vi "Count Pattern Frequencies.vi"(10 "Order":i32=1, 11 "File Data Array":T1[](array[typedef])) -> (3 "Pattern Frequencies":map{string[], i32}(c390))   [LabVIEW 2020]
uses:
  <vilib>/Utility/miscctls.llb/LVMapReplaceAction.ctl
  File Metadata.ctl
  Node.ctl
  Source to Sink Array.ctl
  File Data.ctl
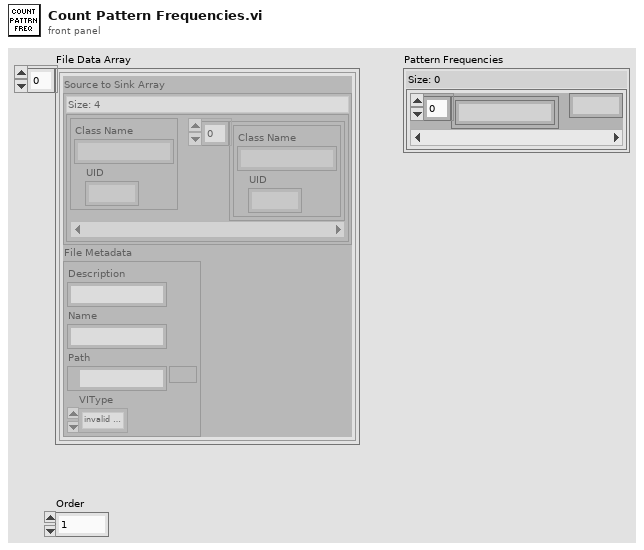
[diagram p1: front panel]
types:
  T1 = typedef "File Data.ctl" = cluster{"Source to Sink Array":T2, "File Metadata":T4}
  T2 = typedef "Source to Sink Array.ctl" = map{T3, T3[]}
  T3 = typedef "Node.ctl" = cluster{"Class Name":string, "UID":i32}
  T4 = typedef "File Metadata.ctl" = cluster{"Description":string, "Name":string, "Path":path, "VIType":enum32{"invalid VI type", "Standard VI", "Control VI", "Global VI", "Polymorphic VI", "Configuration VI", "SubSystem", "Facade VI", "Method VI", "Statechart Diagram VI"}}
  T5 = typedef "LVMapReplaceAction.ctl" = enum32{"Modify Entry only if found", "Add or Modify Entry", "Delete Entry"}
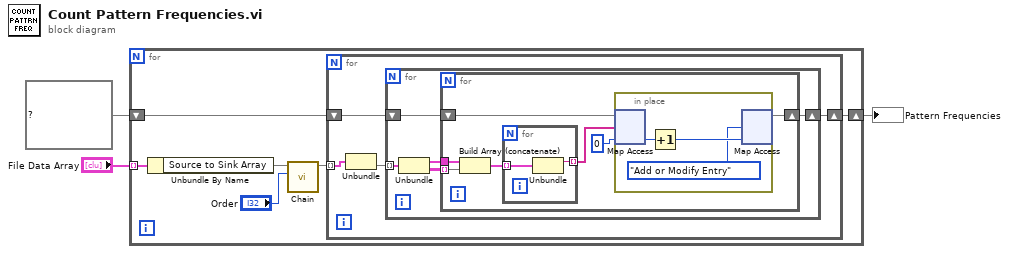
[diagram p0: block diagram]
diagram:
  n1 = for {
    shift-right: [w8] -> w3
    shift-left: map{string[], i32} {} ("Pattern Frequencies") -> [w9]
    tunnel: "File Data Array" -> [w5] mode=indexing
    n2 = Unbundle By Name(w5) -> ("Source to Sink Array"=w4:T2)
    n3 = call "Chain.vi"("Order"="Order", "Source to Sink Array"=w4) -> ("Node to Order-Length Paths"=w6:map{i32, map{T3, T3[][]}})  [unwired: 9 in]
    n4 = for {
      tunnel: w6 -> [w11] mode=indexing
      shift-right: [w12] -> w8
      shift-left: w9 -> [w13]
      n5 = Unbundle(w11) -> ("Source to Sink Array"=w10:map{T3, T3[][]})  [unwired: 1 out]
      n6 = for {
        tunnel: w10 -> [w18] mode=indexing
        shift-right: [w14] -> w12
        shift-left: w13 -> [w15]
        n7 = Unbundle(w18) -> ("Source"=w17:T3, "Sinks"=w16:T3[][])
        n8 = for {
          tunnel: w17 -> [w25]
          tunnel: w16 -> [w24] mode=indexing
          shift-right: [w19] -> w14
          shift-left: w15 -> [w20]
          n9 = Build Array (concatenate)(w25, w24) -> (w23:T3[])
          n10 = for {
            tunnel: w23 -> [w30] mode=indexing
            tunnel: [w29] -> w22 mode=indexing
            n11 = Unbundle(w30) -> ("Class Name"=w29:string)  [unwired: 1 out]
          }
          n12 = in-place {
            n13 = in-place-map #1(w20, w22, 0) -> (w28:i32)  [unwired: 1 out]
            n14 = Increment(x=w28) -> (x+1=w27:i32)
            n15 = in-place-map #1(w27, LVMapReplaceAction."Add or Modify Entry" ("action")) -> (w19:map{string[], i32})  [unwired: 2 out]
          }
        }
      }
    }
  }
  "Pattern Frequencies" <- w3
